vi "Hide Show.vi"(6 "Controls[]":refnum<vi>[](array[refnum]), 7 "Visible?":bool, 8 "Error In":errorcluster) -> (0 "Error Out":errorcluster)   [LabVIEW 2014]
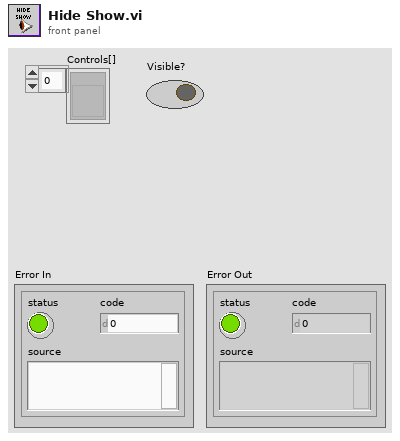
[diagram p1: front panel]
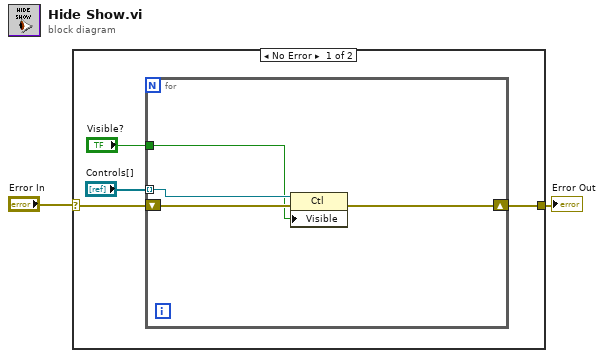
[diagram p0: block diagram]
diagram:
  n1 = case shown="No Error" "Error In" {
    selector: "Error In" -> [w6 w11]
    tunnel: [w4 w11] -> w1
    frame No Error {
      n2 = for {
        shift-right: [w9] -> w4
        shift-left: w6 -> [w10]
        tunnel: "Visible?" -> [w7]
        tunnel: "Controls[]" -> [w8] mode=indexing
        n3 = property class="Ctl"(reference=w8, error in=w10, "Visible"=w7) -> (error out=w9:errorcluster)  [unwired: 1 out]
      }
    }
    frame Error {
    }
  }
  "Error Out" <- w1
